vi "자가진단퀴즈.vi"() -> ()   [LabVIEW 2013]
panel:
  in  "불리언 기본값":bool
  in  "숫자형 기본값":dbl
  in  "케이스 조건":bool
  in  "문자열":string
  out "숫자형":i32
  out "배열 2":i32[](array[numeric])
  out "배열":i32[](array[numeric])
  in  "불리언":bool
  out "인덱싱 비활성화 출력":i32
  out "인덱싱 활성화 출력":i32[](array[numeric])
  # "(1)"
  # "(2)"
  # "(3)"
  # "(4)"
  # "(5)"
  # "(6)"
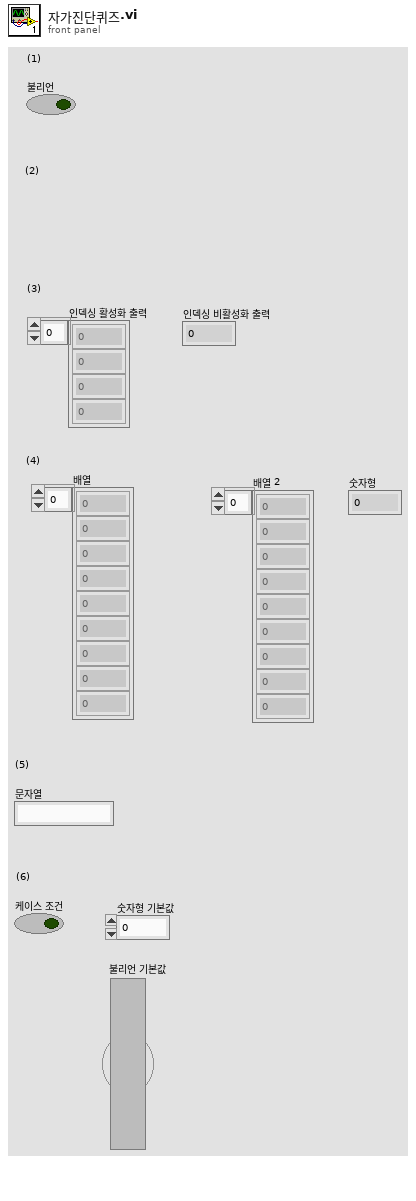
[diagram p1: front panel]
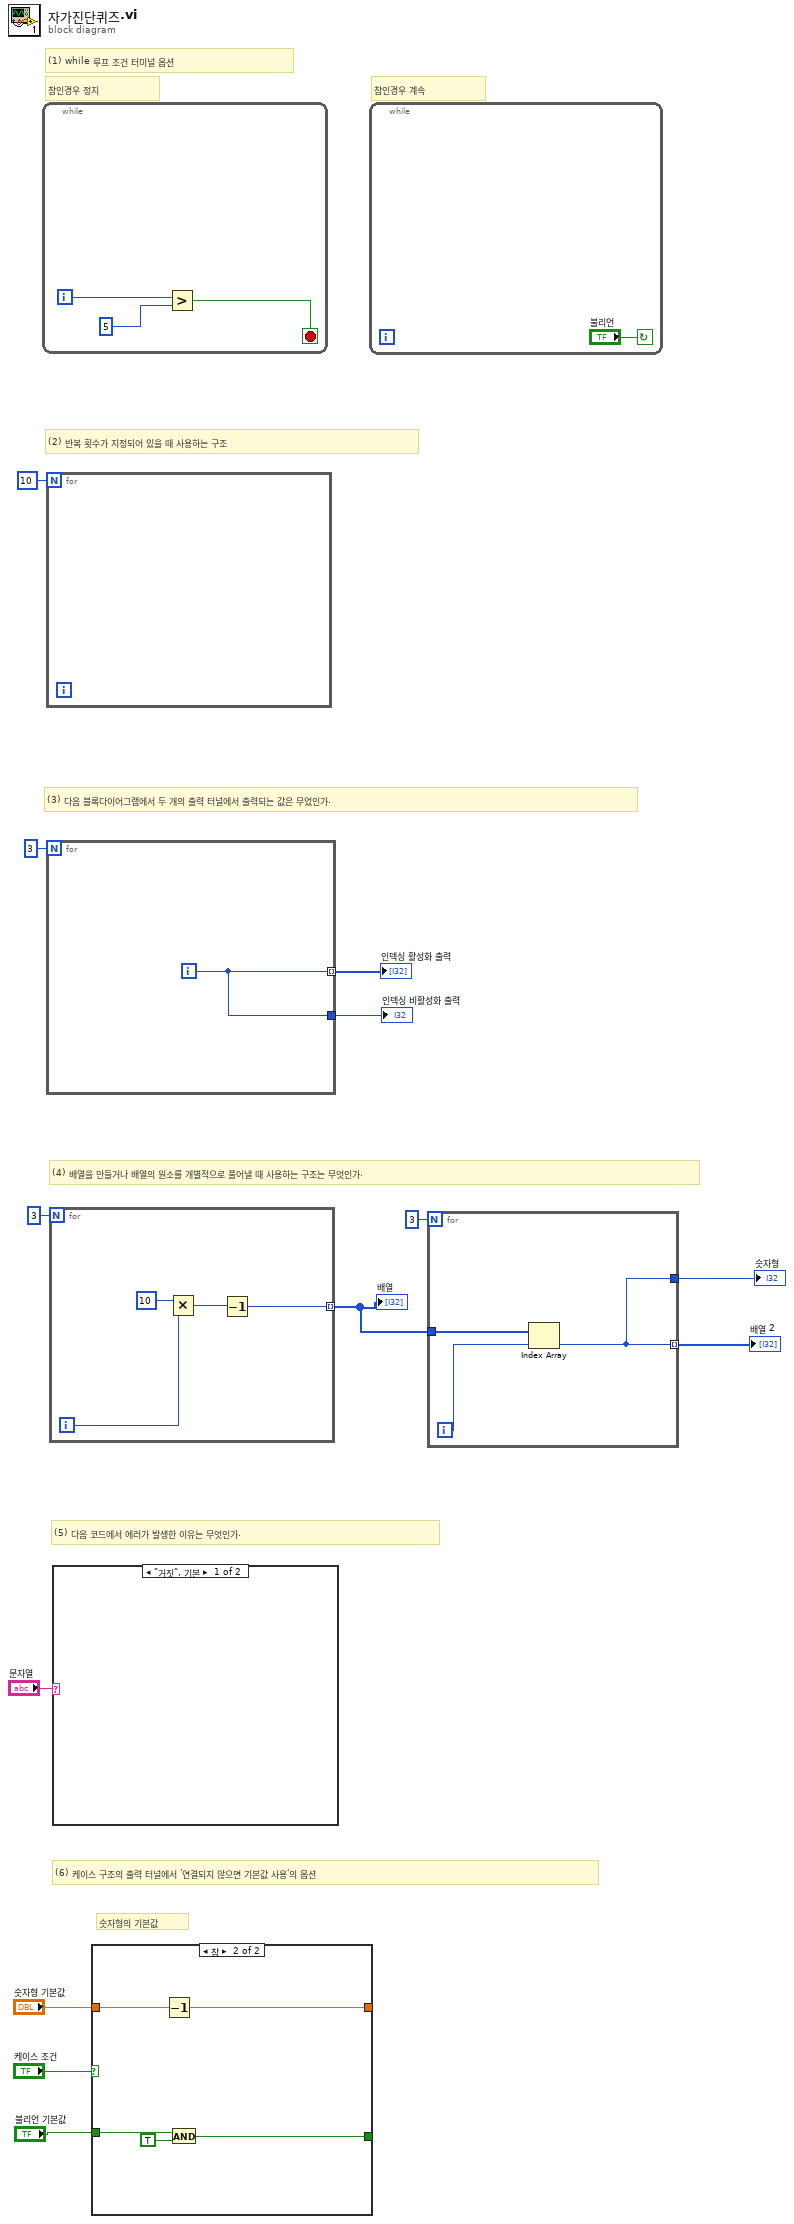
[diagram p0: block diagram]
diagram:
  # "숫자형의 기본값"
  # "(6) 케이스 구조의 출력 터널에서 '연결되지 않으면 기본값 사용'의 옵션"
  # "(5) 다음 코드에서 에러가 발생한 이유는 무엇인가."
  # "(4) 배열을 만들거나 배열의 원소를 개별적으로 풀어낼 때 사용하는 구조는 무엇인가."
  # "(3) 다음 블록다이어그램에서 두 개의 출력 터널에서 출력되는 값은 무었인가."
  # "(2) 반복 횟수가 지정되어 있을 때 사용하는 구조"
  # "참인경우 계속"
  # "참인경우 정지"
  # "(1) while 루프 조건 터미널 옵션"
  n1 = while {
    i -> [w15]
    stop <- w14 stop-if-true
    n2 = Greater?(x=w15, y=5) -> (0:w14:bool)
  }
  n3 = for {
    N: 10 -> [_]
  }
  n4 = for {
    N: 3 -> [_]
    tunnel: [w17] -> w11 mode=indexing
    tunnel: [w17] -> w10
    i -> [w17]
  }
  "인덱싱 활성화 출력" <- w11
  "인덱싱 비활성화 출력" <- w10
  n5 = for {
    N: 3 -> [_]
    tunnel: [w18] -> w5 mode=indexing
    i -> [w20]
    n6 = Multiply(x=10, y=w20) -> (x*y=w19:i32)
    n7 = Decrement(x=w19) -> (x-1=w18:i32)
  }
  "배열" <- w5
  n8 = case shown="\"거짓\", 기본" "문자열" {
    frame "거짓", Default {
    }
    frame "참" {
    }
  }
  n9 = case shown="참" "케이스 조건" {
    tunnel: "숫자형 기본값" -> [_ w26]
    tunnel: [_ w25] -> _
    tunnel: "불리언 기본값" -> [_ w23]
    tunnel: [_ w22] -> _
    frame False {
    }
    frame True {
      n10 = Decrement(x=w26) -> (x-1=w25:dbl)
      n11 = And(x=w23, y=TRUE) -> (x .and. y?=w22:bool)
    }
  }
  n12 = while {
    stop <- "불리언" continue-if-true
  }
  n13 = for {
    N: 3 -> [_]
    tunnel: w5 -> [w30]
    tunnel: [w28] -> w8 mode=indexing
    tunnel: [w28] -> w6
    i -> [w29]
    n14 = Index Array(array=w30, index=w29) -> (element=w28:i32)
  }
  "배열 2" <- w8
  "숫자형" <- w6
